vi "APLUS 4 Wire Unbalanced System.vi"(0 "Modbus Master in":refnum<class "Modbus Master.lvclass">, 1 "Reset WattHours":bool, 2 "Power Input":T2 {"Voltage (V):Element 1 Avg" format="%.3g"; "Voltage (V):Element 2 Avg" format="%.3g"; "Max Watt Hours" format="%.3g"; "Power Factor:Element 2" format="%.3g"; "Power Factor:Element 1" format="%.3g"; "Apparent Power (VA):Element 2" format="%.3g"; "Apparent Power (VA):Element 1" format="%.3g"; "Frequency (Hz):Element 1" format="%.3g"; "Time:Element 1" format="%.3g"; "Voltage Crest Factor:Element 2" format="%.3g"; "Voltage Crest Factor:Element 1" format="%.3g"; "Voltage Harmonic (%):Element 2" format="%.3g"; "Voltage Harmonic (%):Element 1" format="%.3g"; "Current Crest Factor:Element 2" format="%.3g"; "Current Crest Factor:Element 1" format="%.3g"; "Voltage (V):Element 1" format="%.3g"; "Voltage (V):Element 2" format="%.3g"; "Watt Hours (Wh):Sigma" format="%.3f"; "Power (W):Sigma" format="%.3g"; "Current (A):Element 2" format="%.3e"; "Current (A):Element 1" format="%.3e"}, 5 "error in (no error)":errorcluster) -> (8 "Holding Registers":u16[](array[numeric]), 12 "Power":sgl, 14 "Modbus Master out":refnum<class "Modbus Master.lvclass">, 16 "PowerData":T2 {"Voltage (V):Element 1 Avg" format="%.3g"; "Voltage (V):Element 2 Avg" format="%.3g"; "Max Watt Hours" format="%.3g"; "Power Factor:Element 2" format="%.3g"; "Power Factor:Element 1" format="%.3g"; "Apparent Power (VA):Element 2" format="%.3g"; "Apparent Power (VA):Element 1" format="%.3g"; "Frequency (Hz):Element 1" format="%.3g"; "Time:Element 1" format="%.3g"; "Voltage Crest Factor:Element 2" format="%.3g"; "Voltage Crest Factor:Element 1" format="%.3g"; "Voltage Harmonic (%):Element 2" format="%.3g"; "Voltage Harmonic (%):Element 1" format="%.3g"; "Current Crest Factor:Element 2" format="%.3g"; "Current Crest Factor:Element 1" format="%.3g"; "Voltage (V):Element 1" format="%.3g"; "Voltage (V):Element 2" format="%.3g"; "Watt Hours (Wh):Sigma" format="%.3f"; "Power (W):Sigma" format="%.3g"; "Current (A):Element 2" format="%.3e"; "Current (A):Element 1" format="%.3e"}, 19 "error out":errorcluster)   [LabVIEW 2020]
uses:
  <vilib>/NI/Modbus Library/API/Master/Modbus Master.lvclass
  Trunk/Utility/Type Definitions/UTILITY Power Data.ctl
  Type Definitions/APLUS Commands.ctl
panel:
  in  "Voltage (L2-N)":T1=103 items=["L1 Voltage (V) -14"=99, "L1 Voltage (V) -4U"=101, "L2 Voltage (V) -4U"=103, "L1 RMS Current (Amps) -14"=115, "L1 RMS Current (Amps) -4U"=117, "L2 RMS Current (Amps) -4U"=119, "Frequency (Hz) -All"=157, "Sys Power (Watts)-14"=133, "L1 Power (Watts)-4U"=135, "L2 Power (Watts)-4U"=137, "L1 Power Factor-14"=159, "L1 Power Factor-4U"=161, "L2 Power Factor-4U"=163, "L1 Apparent Power (VA)-14"=149, "L1 Apparent Power (VA)-4U"=151, "L2 Apparent Power (VA)-4U"=153, "Voltage Total Harmonic Distortion (%)-All"=235, "Active Energy Incoming-14"=1579, "Unit Factor-14"=1627, "Remainder Active Energy Incoming-14"=5999, "System Type"=2199]
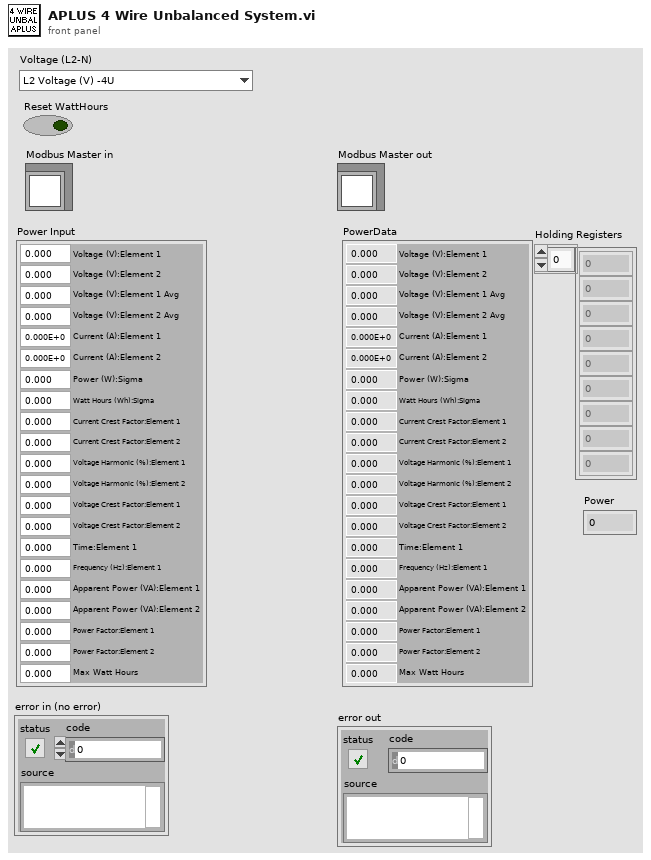
[diagram p1: front panel]
types:
  T1 = typedef "APLUS Commands.ctl" = u16
  T2 = typedef "UTILITY Power Data.ctl" = cluster{"Current (A):Element 1":dbl, "Current (A):Element 2":dbl, "Power (W):Sigma":dbl, "Watt Hours (Wh):Sigma":dbl, "Voltage (V):Element 2":dbl, "Voltage (V):Element 1":dbl, "Current Crest Factor:Element 1":dbl, "Current Crest Factor:Element 2":dbl, "Voltage Harmonic (%):Element 1":dbl, "Voltage Harmonic (%):Element 2":dbl, "Voltage Crest Factor:Element 1":dbl, "Voltage Crest Factor:Element 2":dbl, "Time:Element 1":dbl, "Frequency (Hz):Element 1":dbl, "Apparent Power (VA):Element 1":dbl, "Apparent Power (VA):Element 2":dbl, "Power Factor:Element 1":dbl, "Power Factor:Element 2":dbl, "Max Watt Hours":dbl, "Voltage (V):Element 2 Avg":dbl, "Voltage (V):Element 1 Avg":dbl}
  T3 = typedef "Wago Voltage Range Selector.ctl" = enum16{"Off", "115V 60Hz", "230V 60Hz", "100V 50Hz", "230V 50Hz"}
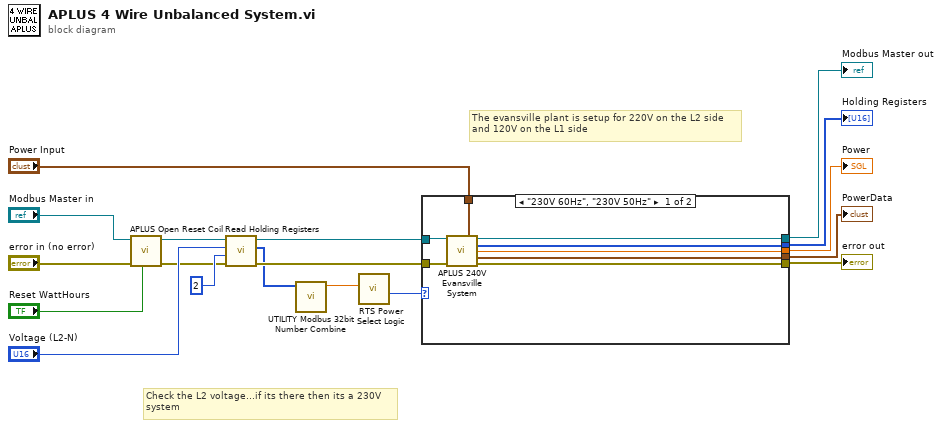
[diagram p0: block diagram]
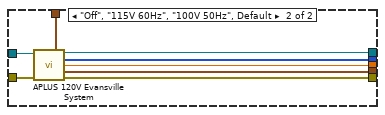
[diagram p2: hidden frame]
diagram:
  # "Check the L2 voltage...if its there then its a 230V\nsystem"
  # "The evansville plant is setup for 220V on the L2 side\nand 120V on the L1 side"
  n1 = call "APLUS Open Reset Coil.vi"("Reset WattHours"="Reset WattHours", "error in (no error)"="error in (no error)", "Modbus Master in"="Modbus Master in") -> ("error out"=w7:errorcluster, "Modbus Master out"=w5:refnum<class "Modbus Master.lvclass">)  [unwired: 7 in]
  n2 = call-dynamic "Read Holding Registers.vi"("error in"=w7, "number of inputs"=u16 2 ("Quantity"), "starting address"="Voltage (L2-N)", "Modbus master in"=w5) -> ("error out"=w6:errorcluster, "register values"=w3:u16[], "Modbus master out"=w4:refnum<class "Modbus Master.lvclass">)  [unwired: 5 in]
  n3 = call "UTILITY Modbus 32bit Number Combine.vi"("Holding Registers"=w3) -> ("Data"=w2:sgl)  [unwired: 9 in, 1 out]
  n4 = call "RTS Power Select Logic.vi"("Voltage in"=w2) -> ("Voltage Range Selector 1"=w1:T3)  [unwired: 8 in, 2 out]
  n5 = case shown="\"230V 60Hz\", \"230V 50Hz\"" w1 {
    tunnel: "Power Input" -> [w19 w34]
    tunnel: [w22 w33] -> w14
    tunnel: [w23 w32] -> w13
    tunnel: [w24 w31] -> w12
    tunnel: [w21 w30] -> w11
    tunnel: [w25 w29] -> w10
    tunnel: w6 -> [w26 w28]
    tunnel: w4 -> [w20 w27]
    frame "230V 60Hz", "230V 50Hz" {
      n6 = call "APLUS 240V Evansville System.vi"("Modbus Master in"=w20, "Power Input"=w19, "error in (no error)"=w26) -> ("Modbus Master out"=w21:refnum<class "Modbus Master.lvclass">, "Holding Registers"=w22:u16[], "Power out"=w23:sgl, "PowerData"=w24:T2, "error out"=w25:errorcluster)  [unwired: 8 in]
    }
    frame "Off", "115V 60Hz", "100V 50Hz", Default {
      n7 = call "APLUS 120V Evansville System.vi"("Modbus Master in"=w27, "Power Input"=w34, "error in (no error)"=w28) -> ("Modbus Master out"=w30:refnum<class "Modbus Master.lvclass">, "Holding Registers"=w33:u16[], "Power out"=w32:sgl, "PowerData"=w31:T2, "error out"=w29:errorcluster)  [unwired: 8 in]
    }
  }
  "Holding Registers" <- w14
  "Power" <- w13
  "Modbus Master out" <- w11
  "error out" <- w10
  "PowerData" <- w12
